vi "Read Var Access.vi"(8 "error in (no error)":errorcluster, 11 "Var Bus in":refnum<class "Var Bus.lvclass">) -> (0 "error out":errorcluster, 2 "Var Access":refnum<class "Var_Access.lvclass">[](array[class]), 3 "Var Bus out":refnum<class "Var Bus.lvclass">)   [LabVIEW 2021, in "Var Bus.lvclass"]
uses:
  Var Bus.lvclass
  Var Access/Var_Access.lvclass
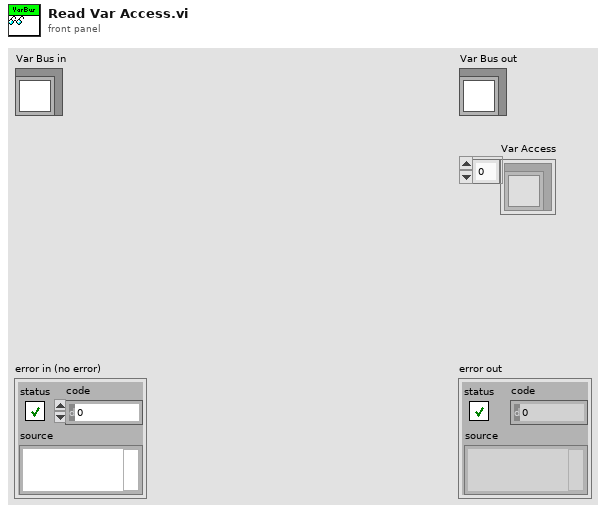
[diagram p1: front panel]
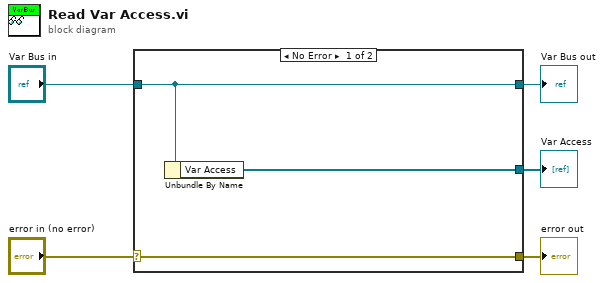
[diagram p0: block diagram]
diagram:
  n1 = case shown="No Error" "error in (no error)" {
    selector: "error in (no error)" -> [w8 w9]
    tunnel: [w8 w9] -> w4
    tunnel: [w7 w10] -> w2
    tunnel: "Var Bus in" -> [w7 w10]
    tunnel: [w6 _] -> w1
    frame No Error {
      n2 = Unbundle By Name(w7) -> ("Var Access"=w6:refnum<class "Var_Access.lvclass">[])
    }
    frame Error {
    }
  }
  "error out" <- w4
  "Var Bus out" <- w2
  "Var Access" <- w1
